vi "Test Serial.vi"() -> ()   [LabVIEW 2014]
uses:
  FPGA/RS485 In.ctl
  Devices/Vaisala Probe/FPGA Interface/FPGA Vaisala.lvclass
  Devices/Vaisala Probe/Vaisala.lvclass/Vaisala.ctl
  Devices/Vaisala Probe/FPGA Interface/FPGA Vaisala.lvclass/FPGA Vaisala.ctl
  Devices/Vaisala Probe/Accessors/Write Address.vi
  Devices/Vaisala Probe/FPGA Interface/Accessors/Write FPGA Ref.vi
  <vilib>/FPGAPlugInAG/cRIO-9081/niLvFpga_Open_cRIO-9081.vi
  <vilib>/Utility/error.llb/Error Cluster From Error Code.vi
  <vilib>/rvi/errors/niLvFpgaAdjustHostInterfaceError.vi
  <vilib>/RVI Host/nirviSupport.llb/nirviErrorClusterFromErrorCode.vi
  <vilib>/FPGAPlugInAG/cRIO-9081/niLvFpga_Close_cRIO-9081.vi
  <vilib>/rvi/interface/nirviOpenFPGA/nirviOpenFPGA.xnode
  <vilib>/rvi/interface/nirviReadWriteControl/nirviReadWriteControl.xnode
  <vilib>/rvi/interface/nirviMethod/nirviMethod.xnode
  <vilib>/rvi/interface/nirviCloseFPGA/nirviCloseFPGA.xnode
  NiFpgaLv.dll
  <vilib>/FPGAPlugInAG/cRIO-9081/niLvFpga_AcknowledgeIrq_cRIO-9081.vi
  <vilib>/rvi/interface/nirviMethod/StockFPGA_InlinedMethodWaitForSingleIRQ.vi
  <vilib>/FPGAPlugInAG/cRIO-9081/niLvFpga_WaitOnIrq_cRIO-9081.vi
  Devices/Vaisala Probe/Vaisala.lvclass
panel:
  in  "Write Port":T1(ring)=enum."Port 2"
  in  "Read Port":T1(ring)=enum."Port 2"
  in  "Write 1x":bool
  in  "read 1x":bool
  in  "String":string="send 1"
  out "string":string
  in  "Read Timeout (ms)":i32=1
  out "Output":T2={"Data"=[0, 0, 0, 0, 0, 0, 0, 0, 0, 0, 0, 0, 0, 0, 0, 0, 0, 0, 0, 0, 0, 0, 0, 0, 0, 0, 0, 0, 0, 0, 0, 0, 0, 0, 0, 0, 0, 0, 0, 0, 0, 0, 0, 0, 0, 0, 0, 0, 0, 0, 0, 0, 0, 0, 0, 0, 0, 0, 0, 0, 0, 0, 0, 0, 0, 0, 0, 0, 0, 0, 0, 0, 0, 0, 0, 0, 0, 0, 0, 0, 0, 0, 0, 0, 0, 0, 0, 0, 0, 0, 0, 0, 0, 0, 0, 0, 0, 0, 0, 0], "NumBytes"=0, "RS485_Cmd"=enum."Read", "New"=FALSE, "Port"=enum."Port 1", "Timeout (ms)"=0}
  in  "Write Timeout":i32=1
  in  "Wait":u32=10
  in  "read":bool
  in  "Write":bool
  out "current time":timestamp
  in  "Stop":bool
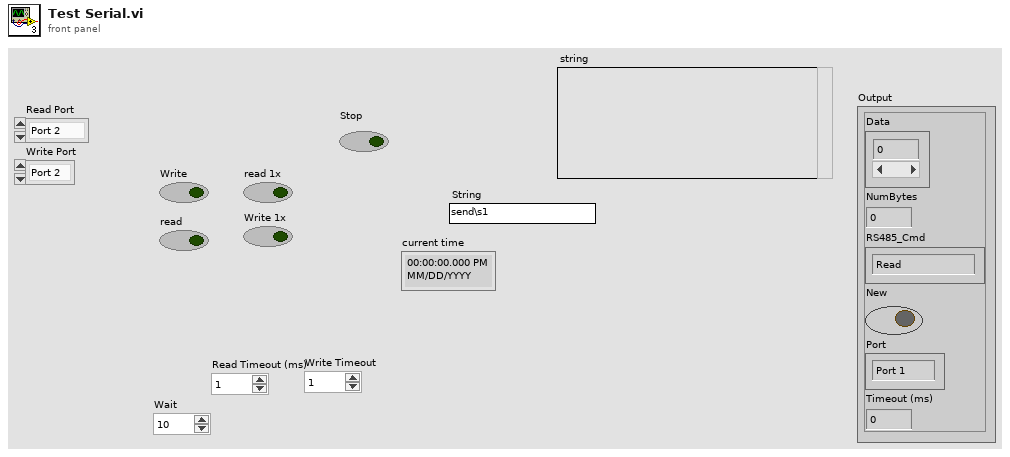
[diagram p1: front panel]
types:
  T1 = enum16{"Port 1", "Port 2", "Port 3", "Port 4", "None"}
  T2 = typedef "RS485 In.ctl" = cluster{"Data":u8[], "NumBytes":i32, "RS485_Cmd":enum16{"Read", "Write", "Idle"}, "New":bool, "Port":enum16{"Port 1", "Port 2", "Port 3", "Port 4", "None"}, "Timeout (ms)":i32}
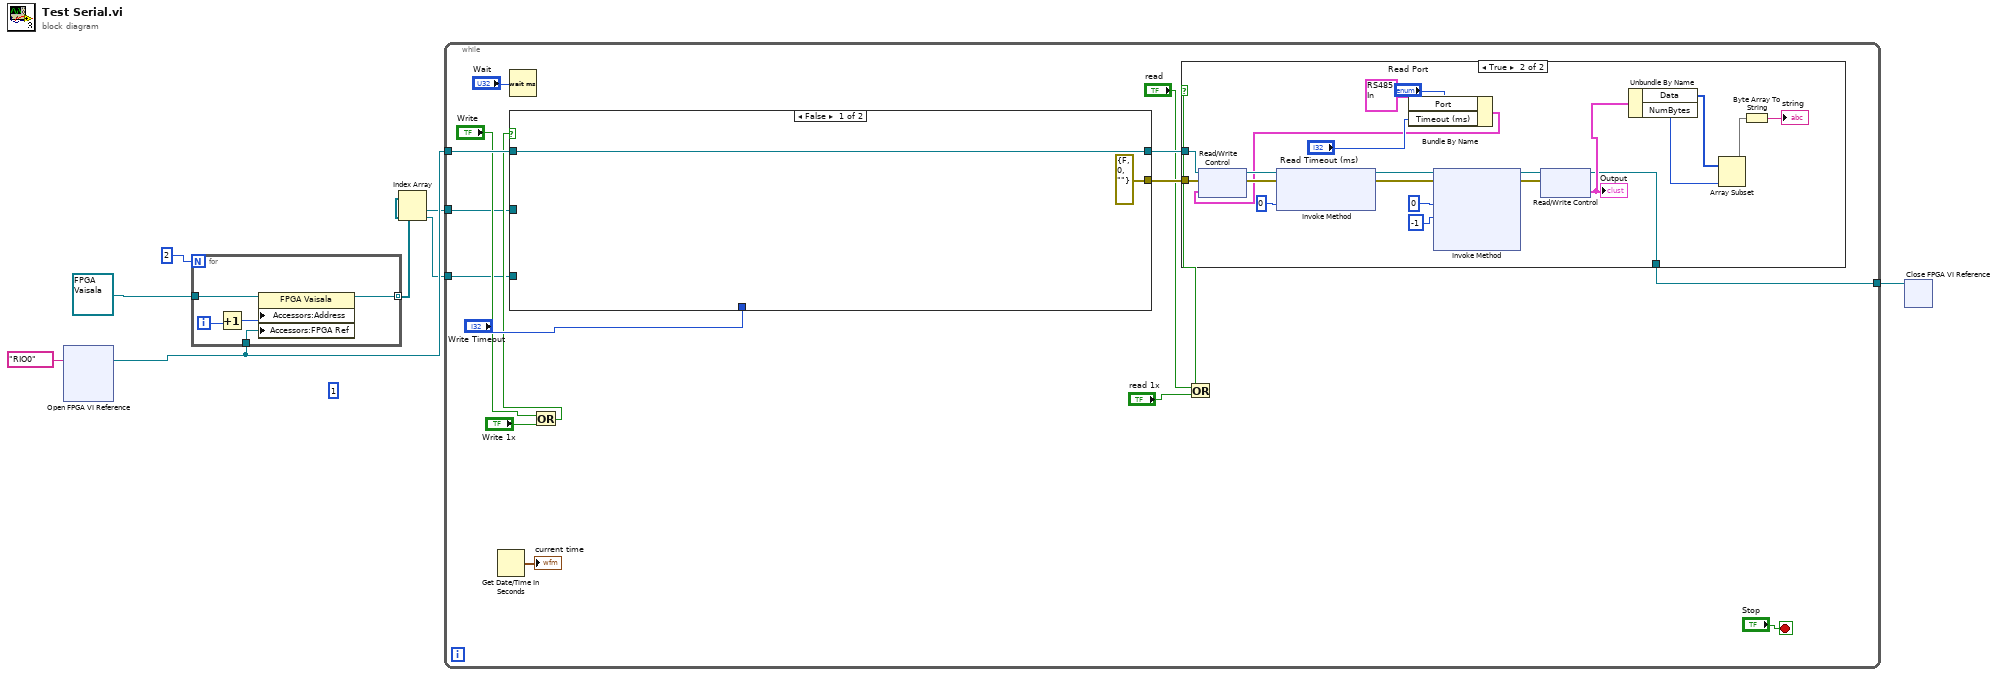
[diagram p0: block diagram]
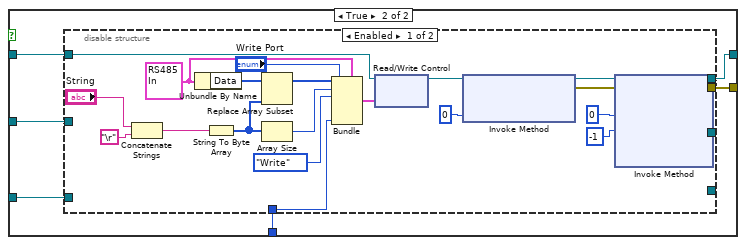
[diagram p3: hidden frame]
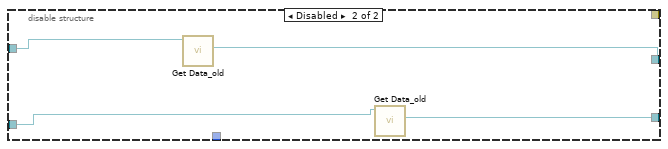
[diagram p4: hidden frame]
diagram:
  (unwired) u8 1 ("Address")
  n1 = xnode "Open FPGA VI Reference"("resource name"=tag "RIO0") -> ("FPGA VI Reference Out"=w4:refnum<k20>)  [unwired: 1 in, 1 out]
  n2 = for {
    N: 2 -> [_]
    tunnel: refnum<class "FPGA Vaisala.lvclass"> refnum ("FPGA Vaisala") -> [w13]
    tunnel: w4 -> [w10]
    tunnel: [w9] -> w2 mode=indexing
    i -> [w12]
    n3 = Increment(x=w12) -> (x+1=w11:i32)
    n4 = property class="FPGA Vaisala"(reference=w13, "Accessors:Address"=w11, "Accessors:FPGA Ref"=w10) -> (reference out=w9:refnum<class "FPGA Vaisala.lvclass">)  [unwired: 1 in, 1 out]
  }
  n5 = Index Array(array=w2) -> (element #1=w3:refnum<class "FPGA Vaisala.lvclass">, element #2=w1:refnum<class "FPGA Vaisala.lvclass">)  [unwired: 2 in]
  n6 = while {
    tunnel: w4 -> [w23]
    tunnel: [w22] -> w7
    tunnel: w3 -> [w15]
    tunnel: w1 -> [w14]
    stop <- "Stop" stop-if-true
    n7 = Get Date/Time In Seconds() -> (seconds since 1Jan1904=→"current time":timestamp)
    n8 = Wait (ms)(milliseconds to wait="Wait") -> ()  [unwired: 1 out]
    n9 = Or(x="Write", y="Write 1x") -> (x .or. y?=w16:bool)
    n10 = case shown="False" w16 {
      tunnel: w23 -> [w53 w59]
      tunnel: [w53 w58] -> w28
      tunnel: [errorcluster {"status"=FALSE, "code"=0, "source"=""} ("error out") w57] -> w27
      tunnel: "Write Timeout" -> [_ w56]
      tunnel: w15 -> [_ w55]
      tunnel: w14 -> [_ w54]
      frame False {
      }
      frame True {
        n11 = disable-structure shown="Enabled" {
          disable-tunnel: w59 -> [w80 _]
          disable-tunnel: [w65 _] -> w58
          disable-tunnel: [w64 _] -> w57
          disable-tunnel: w56 -> [w61 _]
          disable-tunnel: w55 -> [_ w84]
          disable-tunnel: [_ w83] -> _
          disable-tunnel: w54 -> [_ w82]
          disable-tunnel: [_ w81] -> _
          frame Enabled {
            w67 = T2 {"Data"=[0, 0, 0, 0, 0, 0, 0, 0, 0, 0, 0, 0, 0, 0, 0, 0, 0, 0, 0, 0, 0, 0, 0, 0, 0, 0, 0, 0, 0, 0, 0, 0, 0, 0, 0, 0, 0, 0, 0, 0, 0, 0, 0, 0, 0, 0, 0, 0, 0, 0, 0, 0, 0, 0, 0, 0, 0, 0, 0, 0, 0, 0, 0, 0, 0, 0, 0, 0, 0, 0, 0, 0, 0, 0, 0, 0, 0, 0, 0, 0, 0, 0, 0, 0, 0, 0, 0, 0, 0, 0, 0, 0, 0, 0, 0, 0, 0, 0, 0, 0], "NumBytes"=0, "RS485_Cmd"=enum."Write", "New"=TRUE, "Port"=enum."Port 3", "Timeout (ms)"=0} ("Input")
            n12 = Concatenate Strings("String", "\r") -> (w72:string)
            n13 = Unbundle By Name(w67) -> ("Data"=w62:u8[])
            n14 = String To Byte Array(string=w72) -> (unsigned byte array=w69:u8[])
            n15 = Replace Array Subset(array=w62, new element=w69) -> (w68:u8[])  [unwired: 1 in]
            n16 = Array Size(array=w69) -> (size(s)=w70:i32)
            n17 = Bundle(cluster=w67, "Data"=w68, "NumBytes"=w70, "RS485_Cmd"=enum16{"Read", "Write", "Idle"}."Write", "Port"="Write Port", "Timeout (ms)"=w61) -> (w66:T2)  [unwired: 1 in]
            n18 = xnode "Read/Write Control"("FPGA VI Reference In"=w80, "Input"=w66) -> ("FPGA VI Reference Out"=w79:refnum<k20>)  [unwired: 1 in, 1 out]
            n19 = xnode "Invoke Method"("FPGA VI Reference In"=w79, "IRQ Number(s)"=0) -> ("FPGA VI Reference Out"=w77:refnum<k20>, "error out"=w76:errorcluster)  [unwired: 1 in]
            n20 = xnode "Invoke Method"("FPGA VI Reference In"=w77, "error in"=w76, "IRQ Number(s)"=0, "Timeout (ms)"=-1) -> ("FPGA VI Reference Out"=w65:refnum<k20>, "error out"=w64:errorcluster)  [unwired: 2 out]
          }
          frame Disabled {
            n21 = call "Get Data_old.vi"("Vaisala Probe in"=w84) -> ("Data Out"=w83:refnum<class "Single_Array.lvclass">)  [unwired: 8 in, 2 out]
            n22 = call "Get Data_old.vi"("Vaisala Probe in"=w82) -> ("Data Out"=w81:refnum<class "Single_Array.lvclass">)  [unwired: 8 in, 2 out]
          }
        }
      }
    }
    n23 = Or(x="read", y="read 1x") -> (x .or. y?=w19:bool)
    n24 = case shown="True" w19 {
      tunnel: w28 -> [w30 w51]
      tunnel: w27 -> [_ w50]
      tunnel: [w30 w32] -> w22
      frame False {
      }
      frame True {
        n25 = Bundle By Name(cluster=T2 {"Data"=[0, 0, 0, 0, 0, 0, 0, 0, 0, 0, 0, 0, 0, 0, 0, 0, 0, 0, 0, 0, 0, 0, 0, 0, 0, 0, 0, 0, 0, 0, 0, 0, 0, 0, 0, 0, 0, 0, 0, 0, 0, 0, 0, 0, 0, 0, 0, 0, 0, 0, 0, 0, 0, 0, 0, 0, 0, 0, 0, 0, 0, 0, 0, 0, 0, 0, 0, 0, 0, 0, 0, 0, 0, 0, 0, 0, 0, 0, 0, 0, 0, 0, 0, 0, 0, 0, 0, 0, 0, 0, 0, 0, 0, 0, 0, 0, 0, 0, 0, 0], "NumBytes"=0, "RS485_Cmd"=enum."Read", "New"=FALSE, "Port"=enum."Port 2", "Timeout (ms)"=0} ("Input"), "Port"="Read Port", "Timeout (ms)"="Read Timeout (ms)") -> (w38:T2)
        n26 = xnode "Read/Write Control"("FPGA VI Reference In"=w51, "error in"=w50, "Input"=w38) -> ("FPGA VI Reference Out"=w44:refnum<k20>, "error out"=w43:errorcluster)
        n27 = xnode "Invoke Method"("FPGA VI Reference In"=w44, "error in"=w43, "IRQ Number(s)"=0) -> ("FPGA VI Reference Out"=w46:refnum<k20>, "error out"=w47:errorcluster)
        n28 = xnode "Invoke Method"("FPGA VI Reference In"=w46, "error in"=w47, "IRQ Number(s)"=0, "Timeout (ms)"=-1) -> ("FPGA VI Reference Out"=w42:refnum<k20>, "error out"=w41:errorcluster)  [unwired: 2 out]
        n29 = xnode "Read/Write Control"("FPGA VI Reference In"=w42, "error in"=w41) -> ("FPGA VI Reference Out"=w32:refnum<k20>, "Output"=w37:T2)  [unwired: 1 out]
        "Output" <- w37
        n30 = Unbundle By Name(w37) -> ("Data"=w36:u8[], "NumBytes"=w35:i32)
        n31 = Array Subset(array=w36, length=w35) -> (w34:u8[])  [unwired: 1 in]
        n32 = Byte Array To String(unsigned byte array=w34) -> (string=→"string":string)
      }
    }
  }
  n33 = xnode "Close FPGA VI Reference"("FPGA VI Reference In"=w7) -> ()  [unwired: 1 in, 1 out]
